vi "OpenHiSpeedDevice.vi"(3 "error in (no error)":errorcluster, 4 "Location ID":u32, 5 "Device name":string) -> (0 "error out":errorcluster, 1 "Handle":u32, 2 "Result":u32)   [LabVIEW 2010]
uses:
  FTCSPI.dll
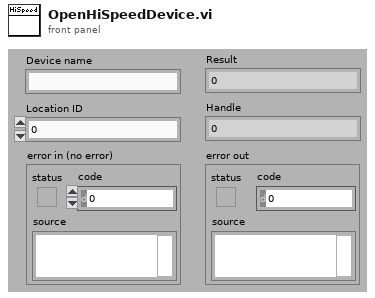
[diagram p1: front panel]
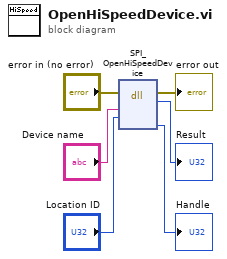
[diagram p0: block diagram]
diagram:
  n1 = dll-call lib="C:/Users/Administrator/Documents/GitHub/labview/FPGA/FTCSPI.dll" fn="SPI_OpenHiSpeedDevice"(error in="error in (no error)", "lpDeviceName"="Device name", "locationId"="Location ID") -> (error out=→"error out":errorcluster, "result"=→"Result":u32, "pftHandle"=→"Handle":u32)  [unwired: 5 in, 1 out]
